vi "test2.vi"() -> ()   [LabVIEW 2013]
panel:
  out "Array 2":string[](array[string])
  out "Array":string[](array[string])
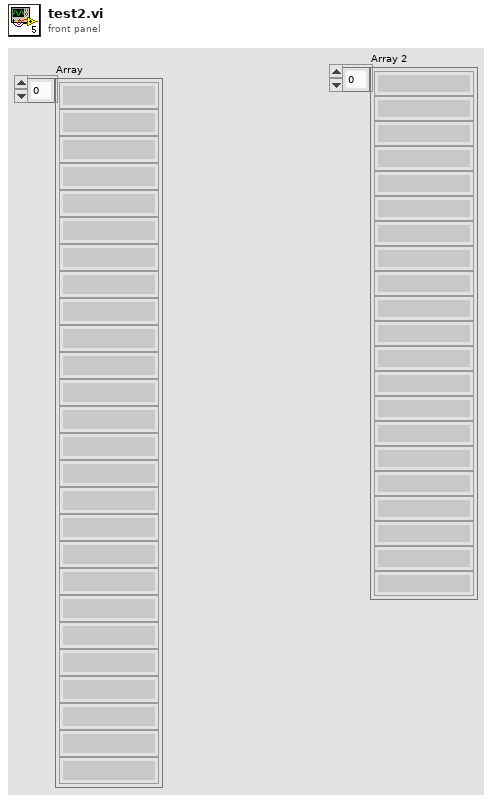
[diagram p1: front panel]
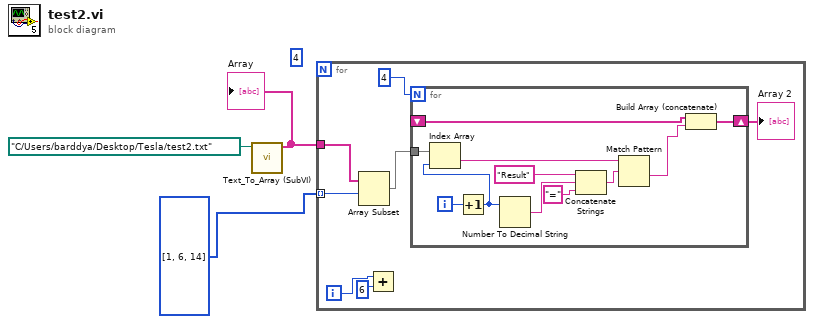
[diagram p0: block diagram]
diagram:
  (unwired) 4
  n1 = call "Text_To_Array (SubVI).vi"("file path"=path "C:/Users/barddya/Desktop/Tesla/test2.txt") -> ("Array"=w2:string[])  [unwired: 9 in, 1 out]
  "Array" <- w2
  n2 = for {
    tunnel: w2 -> [w9]
    tunnel: i32[] [1, 6, 14] -> [w5] mode=indexing
    i -> [w7]
    n3 = Array Subset(array=w9, index=w5) -> (w8:string[])  [unwired: 1 in]
    n4 = Add(x=w7, y=6) -> ()  [unwired: 1 out]
    n5 = for {
      N: 4 -> [_]
      tunnel: w8 -> [w16]
      shift-right: [w12] -> w4
      shift-left: _ -> [w11]
      i -> [w21]
      n6 = Increment(x=w21) -> (x+1=w14:i32)
      n7 = Index Array(array=w16, index=w14) -> (element=w15:string)
      n8 = Number To Decimal String(number=w14) -> (decimal integer string=w18:string)  [unwired: 1 in]
      n9 = Concatenate Strings("Result", w18, "=") -> (w19:string)
      n10 = Match Pattern(string=w15, regular expression=w19) -> (after substring=w13:string)  [unwired: 1 in, 3 out]
      n11 = Build Array (concatenate)(w11, w13) -> (w12:string[])
    }
    "Array 2" <- w4
  }
